vi "run.data_source_type_at.vi"(8 "error in":errorcluster, 11 "Run in":refnum<class "Run.lvclass">) -> (0 "error out":errorcluster, 3 "Run out":refnum<class "Run.lvclass">)   [LabVIEW 2020, in "Run.lvclass"]
doc: "Returns the type (dataset, video, or connection) of the data source attached to the run at the given position."
uses:
  Run.lvclass
  Run.lvclass/Run.ctl
  client.lvlib
panel:
  out "out_type out":i32
  in  "index":i32
  in  "out_type":i32
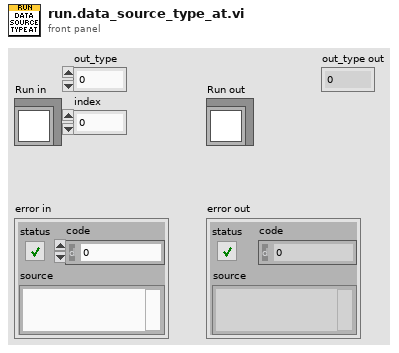
[diagram p1: front panel]
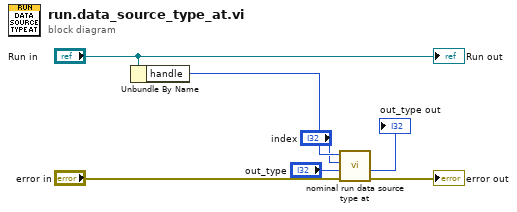
[diagram p0: block diagram]
diagram:
  n1 = Unbundle By Name("Run in") -> ("handle"=w5:i32)
  n2 = call "nominal run data source type at.vi"("error in (no error)"="error in", "out_type"="out_type", "index"="index", "run"=w5) -> ("error out"=→"error out":errorcluster, "out_type out"=→"out_type out":i32)  [unwired: 5 in, 1 out]
  "Run out" <- "Run in"
